vi "AlliGator Enforce Lifetime Positivity.vi"(11 "Constraints in":T1[](array[typedef]) {"Max Value" format="%#.3g"; "Min Value" format="%#.3g"}) -> (3 "Constraints out":T1[](array[typedef]) {"Max Value" format="%#.3g"; "Min Value" format="%#.3g"})   [LabVIEW 2021, in "AlliGator Decay Fit.lvlib"]
doc: "Constrains lifetime parameters to be positive (replacing them by zero otherwise)."
uses:
  AlliGator Decay Fit.lvlib
  AlliGator Decay Fit Parameter Constraints 2.ctl
  Fits/IRF(X)PSED/Decay Fit Parameters In List.ctl
  Fits/Fits.lvlib
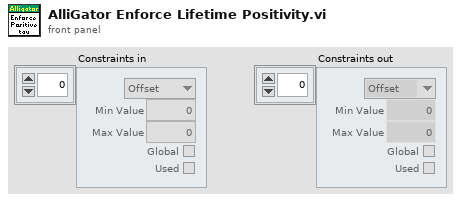
[diagram p1: front panel]
types:
  T1 = typedef "AlliGator Decay Fit.lvlib/AlliGator Decay Fit Parameter Constraints 2.ctl" = cluster{"Fit Parameter":T2, "Min Value":dbl, "Max Value":dbl, "Global":bool, "Used":bool}
  T2 = typedef "Fits.lvlib/Decay Fit Parameters In List.ctl" = enum16{"Offset", "Baseline", "A_1", "tau_1", "A_2", "tau_2"}
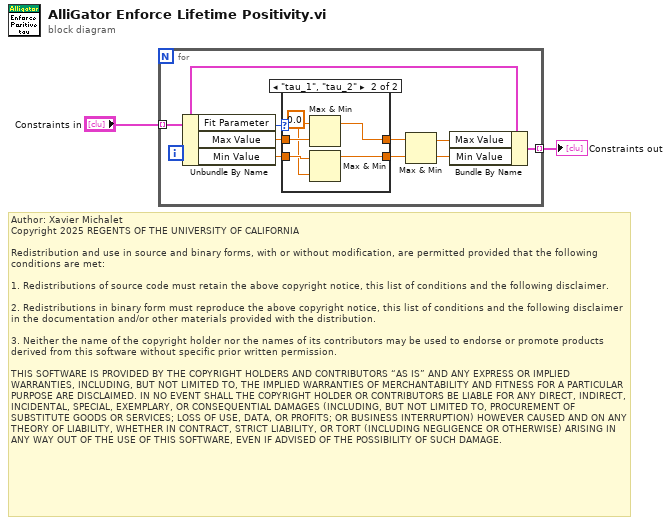
[diagram p0: block diagram]
diagram:
  # "Author: Xavier Michalet\nCopyright 2025 REGENTS OF THE UNIVERSITY OF CALIFORNIA\n\nRedistribution and use in source and binary forms, with or without modification, are permitted provided that the following conditions are met:\n\n1. Redistributions of source code must retain the above copyright notice, this list of conditions and the following disclaimer.\n\n2. Redistributions in binary form must reproduce the above copyright notice, this list of conditions and the following disclaimer in the documentation and/or other materials provided with the distribution.\n\n3. Neither the name of the copyright holder nor the names of its contributors may be used to endorse or promote products derived from this software without specific prior written permission.\n\nTHIS SOFTWARE IS PROVIDED BY THE COPYRIGHT HOLDERS AND CONTRIBUTORS “AS IS” AND ANY EXPRESS OR IMPLIED WARRANTIES, INCLUDING, BUT NOT LIMITED TO, THE IMPLIED WARRANTIES OF MERCHANTABILITY AND FITNESS FOR A PARTICULAR PURPOSE ARE DISCLAIMED. IN NO EVENT SHALL THE COPYRIGHT HOLDER OR CONTRIBUTORS BE LIABLE FOR ANY DIRECT, INDIRECT, INCIDENTAL, SPECIAL, EXEMPLARY, OR CONSEQUENTIAL DAMAGES (INCLUDING, BUT NOT LIMITED TO, PROCUREMENT OF SUBSTITUTE GOODS OR SERVICES; LOSS OF USE, DATA, OR PROFITS; OR BUSINESS INTERRUPTION) HOWEVER CAUSED AND ON ANY THEORY OF LIABILITY, WHETHER IN CONTRACT, STRICT LIABILITY, OR TORT (INCLUDING NEGLIGENCE OR OTHERWISE) ARISING IN ANY WAY OUT OF THE USE OF THIS SOFTWARE, EVEN IF ADVISED OF THE POSSIBILITY OF SUCH DAMAGE."
  n1 = for {
    tunnel: "Constraints in" -> [w9] mode=indexing
    tunnel: [w3] -> w1 mode=indexing
    n2 = Unbundle By Name(w9) -> ("Fit Parameter"=w11:T2, "Max Value"=w10:dbl, "Min Value"=w8:dbl)
    n3 = case shown="\"tau_1\", \"tau_2\"" w11 {
      tunnel: w10 -> [w13 w18]
      tunnel: w8 -> [w12 w17]
      tunnel: [w13 w15] -> w7
      tunnel: [w12 w14] -> w6
      frame "Offset", Default {
      }
      frame "tau_1", "tau_2" {
        w16 = 0.0 ("y")
        n4 = Max & Min(x=w16, y=w18) -> (max(x,y)=w15:dbl)  [unwired: 1 out]
        n5 = Max & Min(x=w17, y=w16) -> (max(x,y)=w14:dbl)  [unwired: 1 out]
      }
    }
    n6 = Max & Min(x=w7, y=w6) -> (max(x,y)=w5:dbl, min(x,y)=w4:dbl)
    n7 = Bundle By Name(cluster=w9, "Max Value"=w5, "Min Value"=w4) -> (w3:T1)
  }
  "Constraints out" <- w1
